vi "HighlightRow.vi"(10 "State":enum16{"InitRows", "GetRows", "LastRow"}(ring), 11 "Script Contents 2":refnum<vi>) -> ()   [LabVIEW 2019, in "Scripts.lvclass"]
uses:
  Scripts.lvclass
  <vilib>/Utility/miscctls.llb/LVRowAndColumnTypeDef.ctl
panel:
  out "Row":dbl
  out "Script Contents":i32(listbox)
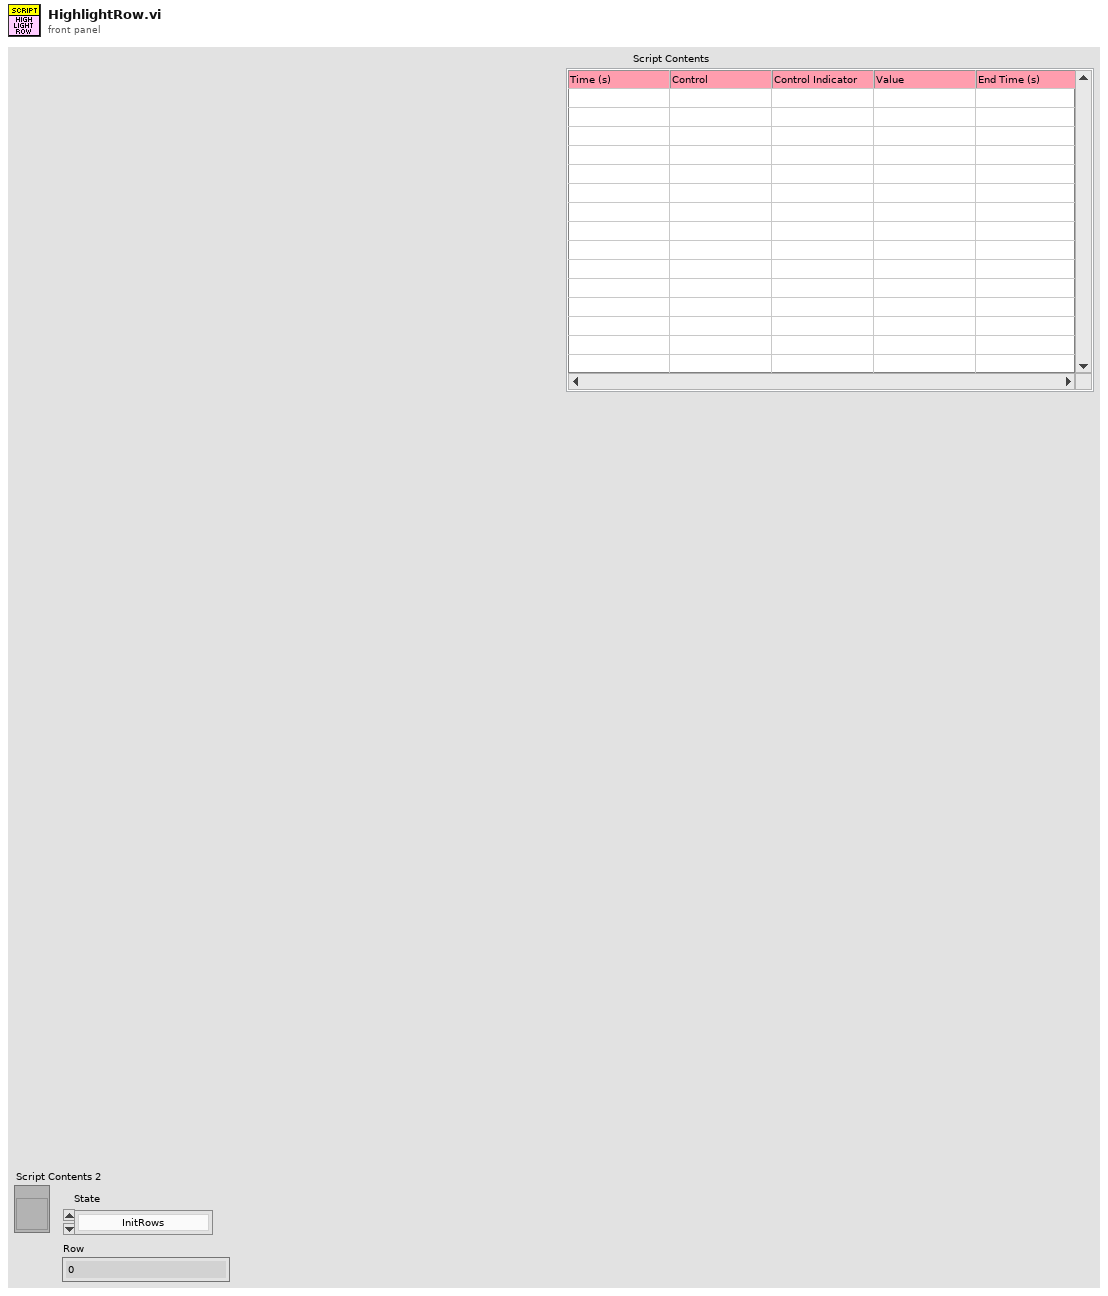
[diagram p1: front panel]
types:
  T1 = typedef "LVRowAndColumnTypeDef.ctl" = cluster{"Row":i32, "Column":i32}
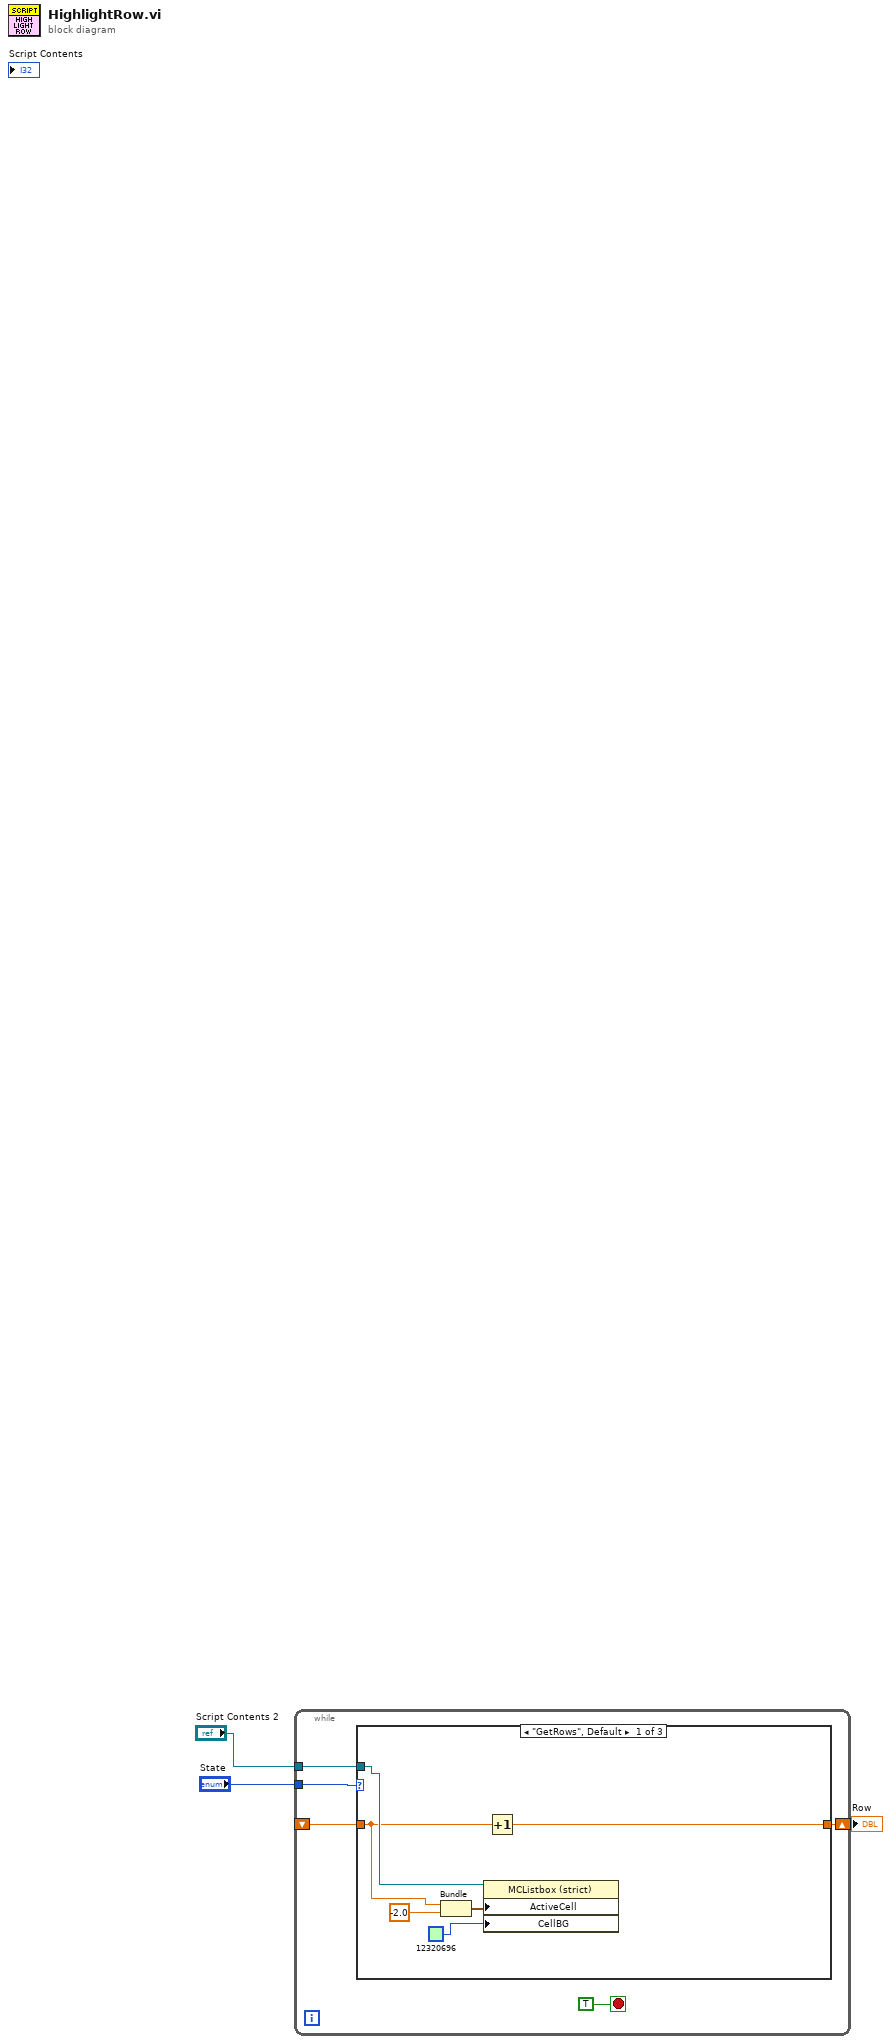
[diagram p0: block diagram]
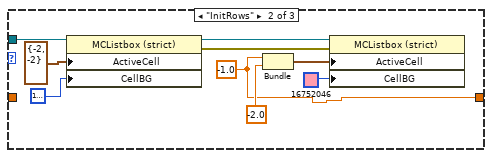
[diagram p2: hidden frame]
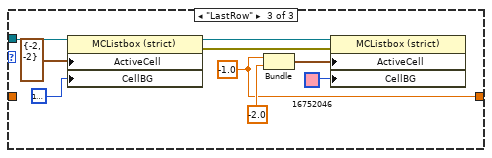
[diagram p3: hidden frame]
diagram:
  n1 = while {
    tunnel: "State" -> [w8]
    shift-right: [w6] -> w2
    shift-left: _ -> [w5]
    tunnel: "Script Contents 2" -> [w4]
    stop <- TRUE stop-if-true
    n2 = case shown="\"GetRows\", Default" w8 {
      tunnel: [w9 w15 w25] -> w6
      tunnel: w5 -> [w10 _ _]
      tunnel: w4 -> [w13 w18 w26]
      frame "GetRows", Default {
        n3 = Bundle(w10, -2.0) -> (w11:cluster{dbl, dbl})  [unwired: 1 in]
        n4 = property on="Property Node" class="MCListbox (strict)"(reference=w13, "ActiveCell"=w11, "CellBG"=u32 12320696) -> ()  [unwired: 1 in, 2 out]
        n5 = Increment(x=w10) -> (x+1=w9:dbl)
      }
      frame "InitRows" {
        w15 = -1.0
        n6 = property on="Property Node" class="MCListbox (strict)"(reference=w18, "ActiveCell"=T1 {"Row"=-2, "Column"=-2} ("Active Cell:Active Cell"), "CellBG"=u32 16777216) -> (reference out=w17:refnum<vi>, error out=w19:errorcluster)  [unwired: 1 in]
        n7 = Bundle(w15, -2.0) -> (w23:cluster{dbl, dbl})  [unwired: 1 in]
        n8 = property on="Property Node" class="MCListbox (strict)"(reference=w17, error in=w19, "ActiveCell"=w23, "CellBG"=u32 16752046) -> ()  [unwired: 2 out]
      }
      frame "LastRow" {
        w25 = -1.0
        n9 = property on="Property Node" class="MCListbox (strict)"(reference=w26, "ActiveCell"=T1 {"Row"=-2, "Column"=-2} ("Active Cell:Active Cell"), "CellBG"=u32 16777216) -> (reference out=w28:refnum<vi>, error out=w29:errorcluster)  [unwired: 1 in]
        n10 = Bundle(w25, -2.0) -> (w32:cluster{dbl, dbl})  [unwired: 1 in]
        n11 = property on="Property Node" class="MCListbox (strict)"(reference=w28, error in=w29, "ActiveCell"=w32, "CellBG"=u32 16752046) -> ()  [unwired: 2 out]
      }
    }
  }
  "Row" <- w2
